vi "FTW-Color-To HSL.vi"(1 "Color":u32(colorbox)) -> (0 "HSL":cluster{"Hue":dbl, "Sat":dbl, "Lum":dbl})   [LabVIEW 2013]
doc: "Converts a 32 bit RGB (Red, Green, Blue) color space value into an HSL (Hue, Saturation, Lumanence) color space value."
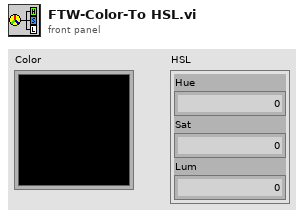
[diagram p1: front panel]
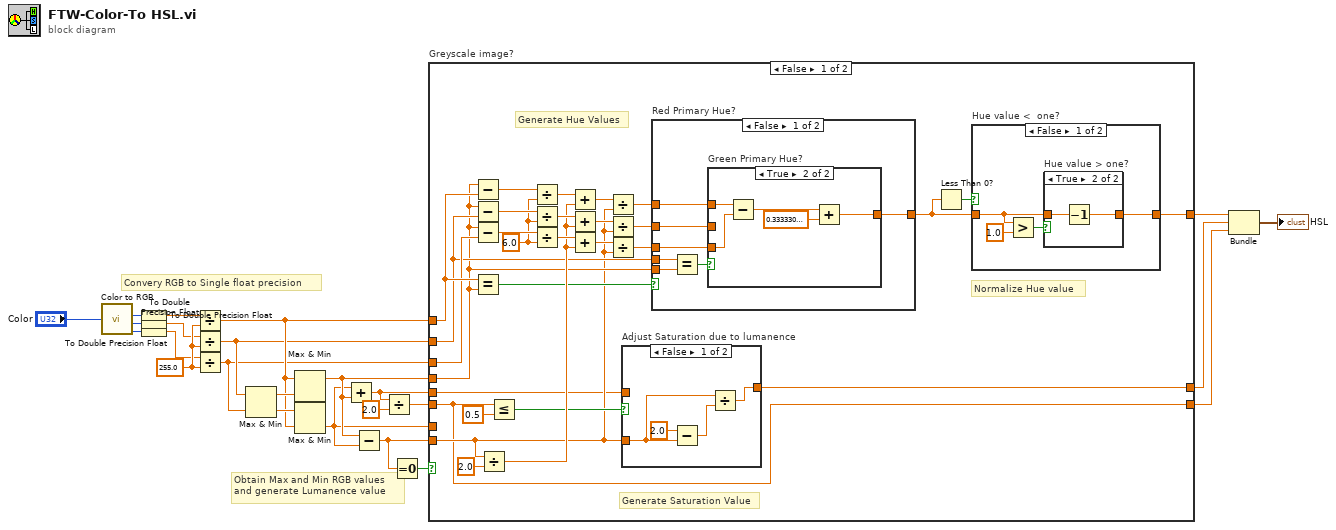
[diagram p0: block diagram]
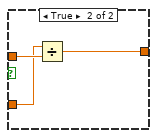
[diagram p2: hidden frame]
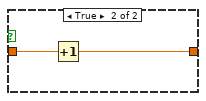
[diagram p4: hidden frame]
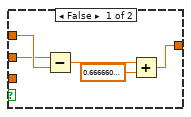
[diagram p5: hidden frame]
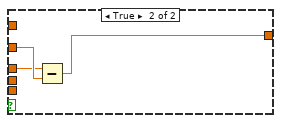
[diagram p6: hidden frame]
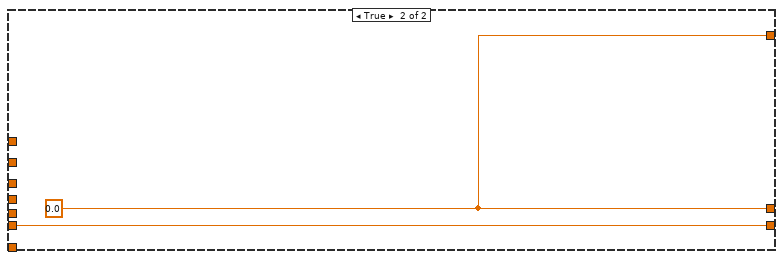
[diagram p7: hidden frame]
diagram:
  w11 = 255.0 ("y")
  # "Convery RGB to Single float precision"
  # "Obtain Max and Min RGB values\nand generate Lumanence value"
  n1 = call <vilib>:"Color to RGB.vi"("Color"="Color") -> ("R"=w17:u8, "G"=w15:u8, "B"=w13:u8)  [unwired: 1 out]
  n2 = To Double Precision Float(number=w17) -> (double precision float=w5:dbl)
  n3 = To Double Precision Float(number=w15) -> (double precision float=w6:dbl)
  n4 = To Double Precision Float(number=w13) -> (double precision float=w7:dbl)
  n5 = Divide(x=w5, y=w11) -> (x/y=w16:dbl)
  n6 = Divide(x=w6, y=w11) -> (x/y=w14:dbl)
  n7 = Divide(x=w7, y=w11) -> (x/y=w12:dbl)
  n8 = Max & Min(x=w14, y=w12) -> (max(x,y)=w23:dbl, min(x,y)=w22:dbl)
  n9 = Max & Min(x=w16, y=w23) -> (max(x,y)=w20:dbl)  [unwired: 1 out]
  n10 = Max & Min(x=w22, y=w16) -> (min(x,y)=w19:dbl)  [unwired: 1 out]
  n11 = Add(x=w19, y=w20) -> (x+y=w8:dbl)
  n12 = Subtract(x=w20, y=w19) -> (x-y=w10:dbl)
  n13 = Divide(x=w8, y=2.0) -> (x/y=w18:dbl)
  n14 = Equal To 0?(x=w10) -> (x = 0?=w9:bool)
  n15 = case "Greyscale image?" shown="False" w9 {
    tunnel: w20 -> [w29 _]
    tunnel: w19 -> [_ _]
    tunnel: w18 -> [w25 w90]
    tunnel: w12 -> [w36 _]
    tunnel: w14 -> [w35 _]
    tunnel: w16 -> [w37 _]
    tunnel: w10 -> [w28 _]
    tunnel: [w32 w91] -> w4
    tunnel: w8 -> [w27 _]
    tunnel: [w26 w91] -> w3
    tunnel: [w25 w90] -> w2
    frame False {
      w42 = 6.0 ("y")
      # "Normalize Hue value"
      # "Generate Hue Values"
      # "Generate Saturation Value"
      n16 = Subtract(x=w29, y=w37) -> (x-y=w53:dbl)
      n17 = Subtract(x=w29, y=w35) -> (x-y=w52:dbl)
      n18 = Subtract(x=w29, y=w36) -> (x-y=w51:dbl)
      n19 = Equal?(x=w37, y=w29) -> (x = y?=w41:bool)
      n20 = Divide(x=w28, y=2.0) -> (x/y=w43:dbl)
      n21 = Less Or Equal?(x=w25, y=0.5) -> (x <= y?=w31:bool)
      n22 = Divide(x=w53, y=w42) -> (x/y=w49:dbl)
      n23 = Divide(x=w52, y=w42) -> (x/y=w48:dbl)
      n24 = Divide(x=w51, y=w42) -> (x/y=w47:dbl)
      n25 = Add(x=w49, y=w43) -> (x+y=w44:dbl)
      n26 = Add(x=w48, y=w43) -> (x+y=w45:dbl)
      n27 = Add(x=w47, y=w43) -> (x+y=w46:dbl)
      n28 = Divide(x=w44, y=w28) -> (x/y=w38:dbl)
      n29 = Divide(x=w45, y=w28) -> (x/y=w39:dbl)
      n30 = Divide(x=w46, y=w28) -> (x/y=w40:dbl)
      n31 = case "Adjust Saturation due to lumanence" shown="False" w31 {
        tunnel: w28 -> [w55 w59]
        tunnel: w27 -> [_ w60]
        tunnel: [w54 w58] -> w26
        frame False {
          n32 = Subtract(x=2.0, y=w55) -> (x-y=w56:dbl)
          n33 = Divide(x=w55, y=w56) -> (x/y=w54:dbl)
        }
        frame True {
          n34 = Divide(x=w59, y=w60) -> (x/y=w58:dbl)
        }
      }
      n35 = case "Red Primary Hue?" shown="False" w41 {
        tunnel: w40 -> [w71 w88]
        tunnel: w39 -> [w72 w89]
        tunnel: w38 -> [w73 _]
        tunnel: w35 -> [w76 _]
        tunnel: w29 -> [w75 _]
        tunnel: [w70 w87] -> w33
        frame False {
          n36 = Equal?(x=w76, y=w75) -> (x = y?=w74:bool)
          n37 = case "Green Primary Hue?" shown="True" w74 {
            tunnel: w73 -> [w81 w86]
            tunnel: w72 -> [w77 _]
            tunnel: w71 -> [_ w85]
            tunnel: [w78 w82] -> w70
            frame False {
              n38 = Subtract(x=w77, y=w81) -> (x-y=w80:dbl)
              n39 = Add(x=w80, y=sgl 0.66666) -> (x+y=w78:dbl)
            }
            frame True {
              n40 = Subtract(x=w86, y=w85) -> (x-y=w84:dbl)
              n41 = Add(x=w84, y=0.3333300054073334) -> (x+y=w82:dbl)
            }
          }
        }
        frame True {
          n42 = Subtract(x=w88, y=w89) -> (x-y=w87:dbl)
        }
      }
      n43 = Less Than 0?(x=w33) -> (x < 0?=w34:bool)
      n44 = case "Hue value <  one?" shown="False" w34 {
        tunnel: w33 -> [w61 w69]
        tunnel: [w62 w68] -> w32
        frame False {
          n45 = Greater?(x=w61, y=1.0) -> (0:w63:bool)
          n46 = case "Hue value > one?" shown="True" w63 {
            tunnel: w61 -> [w65 w67]
            tunnel: [w65 w66] -> w62
            frame False {
            }
            frame True {
              n47 = Decrement(x=w67) -> (x-1=w66:dbl)
            }
          }
        }
        frame True {
          n48 = Increment(x=w69) -> (x+1=w68:dbl)
        }
      }
    }
    frame True {
      w91 = sgl 0.0
    }
  }
  n49 = Bundle(w4, w3, w2) -> (→"HSL":cluster{dbl, dbl, dbl})  [unwired: 1 in]
